vi "Update Item.vi"(8 "error in (no error)":errorcluster, 10 "All Data":refnum<class "Data Item.lvclass">[](array[class]), 11 "Element in":refnum<class "Element.lvclass">) -> (0 "error out":errorcluster, 2 "All Data out":refnum<class "Data Item.lvclass">[](array[class]), 3 "Element out":refnum<class "Element.lvclass">)   [LabVIEW 2026, in "VILab.lvlib" / "Element.lvclass"]
uses:
  Element.lvclass
  Data Item/Data Item.lvclass
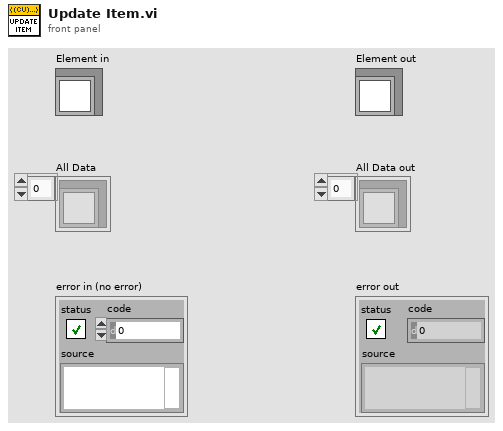
[diagram p1: front panel]
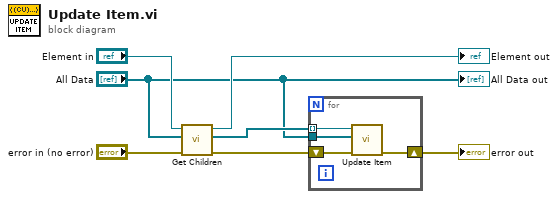
[diagram p0: block diagram]
diagram:
  n1 = call-dynamic "Get Children.vi"("error in (no error)"="error in (no error)", "All Data"="All Data", "Element in"="Element in") -> ("error out"=w5:errorcluster, "Children"=w4:refnum<class "Data Item.lvclass">[], "Element out"=→"Element out":refnum<class "Element.lvclass">)  [unwired: 5 in, 1 out]
  n2 = for {
    shift-right: [w11] -> w7
    shift-left: w5 -> [w10]
    tunnel: w4 -> [w9] mode=indexing
    tunnel: "All Data" -> [w8]
    n3 = call-dynamic "Update Item.vi"("error in (no error)"=w10, "All Data"=w8, "Data Item in"=w9) -> ("error out"=w11:errorcluster)  [unwired: 6 in, 2 out]
  }
  "error out" <- w7
  "All Data out" <- "All Data"
